vi "Test CONNACK packet.vi"() -> ()   [LabVIEW 2013]
uses:
  Control Packets/CONNACK/CONNACK.lvclass
  Control Packets/CONNACK/Connect Return Code -- enum.ctl
  Control Packets/ControlPacket/ControlPacket.lvclass
panel:
  out "error out":errorcluster
  out "Return Code":bool
  out "Packet type":bool
  out "All packets consumed":bool
  out "Complete Packet":bool
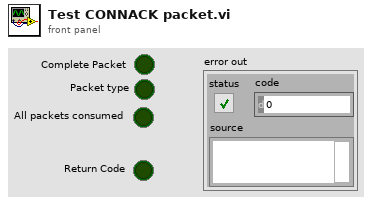
[diagram p1: front panel]
types:
  T1 = typedef "CONNACK.lvclass/Connect Return Code -- enum.ctl" = enum16{"Connection accepted", "Unacceptable protocol version", "Identifier Rejected", "Server Unavailable", "Bad Username or Password", "Not Authorized"}
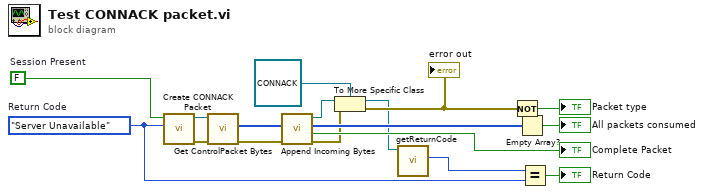
[diagram p0: block diagram]
diagram:
  w6 = FALSE  # Session Present
  w7 = Connect_Return_Code_--_enum."Server Unavailable"  # Return Code
  n1 = call "Create CONNACK Packet.vi"("Return Code"=w7, "Session Present"=w6) -> ("error out"=w3:errorcluster, "CONNACK"=w8:refnum<class "CONNACK.lvclass">)  [unwired: 8 in]
  n2 = call "Get ControlPacket Bytes.vi"("error in (no error)"=w3, "ControlPacket"=w8) -> ("error out"=w2:errorcluster, "Bytes Stream"=w17:u8[])  [unwired: 7 in, 1 out]
  n3 = call "Append Incoming Bytes.vi"("error in (no error)"=w2, "Incoming Packets"=w17) -> ("error out"=w1:errorcluster, "Complete Packet"=→"Complete Packet":bool, "Remaining Packets"=w15:u8[], "ControlPacket"=w13:refnum<class "ControlPacket.lvclass">)  [unwired: 6 in]
  n4 = To More Specific Class(target class=refnum<class "CONNACK.lvclass"> refnum ("CONNACK.lvclass"), reference=w13, error in=w1) -> (specific class reference=w5:refnum<class "CONNACK.lvclass">, error out=w12:errorcluster)
  "error out" <- w12
  n5 = call "getReturnCode.vi"("CONNACK in"=w5) -> ("Return Code"=w4:T1)  [unwired: 8 in, 2 out]
  n6 = Not(x=w12) -> (.not. x?=→"Packet type":bool)
  n7 = Empty Array?(array=w15) -> (empty?=→"All packets consumed":bool)
  n8 = Equal?(x=w4, y=w7) -> (x = y?=→"Return Code":bool)
